vi "Toggle.vi"(1 "Input":bool, 2 "Case":enum16{"Only Press", "Toggle"}(ring)) -> (0 "Output":bool)   [LabVIEW 2014]
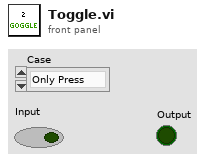
[diagram p1: front panel]
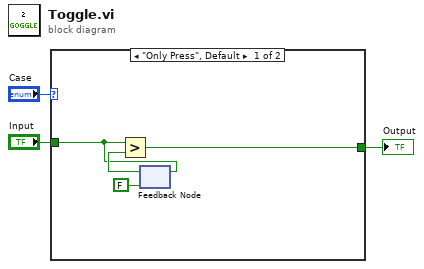
[diagram p0: block diagram]
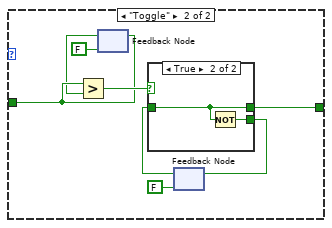
[diagram p2: hidden frame]
diagram:
  n1 = case shown="\"Only Press\", Default" "Case" {
    tunnel: "Input" -> [w5 w12]
    tunnel: [w4 w8] -> w1
    frame "Only Press", Default {
      n2 = feedback #1(FALSE ("A")) -> (w6:bool)
      n3 = Greater?(x=w5, y=w6) -> (0:w4:bool)
      n4 = feedback-in #1(w5) -> ()
    }
    frame "Toggle" {
      n5 = feedback #2(FALSE ("Input")) -> (w11:bool)
      n6 = Greater?(x=w12, y=w11) -> (0:w13:bool)
      n7 = feedback-in #2(w12) -> ()
      n8 = feedback #3(FALSE ("A")) -> (w15:bool)
      n9 = case shown="True" w13 {
        tunnel: w15 -> [w16 w17]
        tunnel: [w16 w18] -> w9
        tunnel: [w16 w17] -> w8
        frame False {
        }
        frame True {
          n10 = Not(x=w17) -> (.not. x?=w18:bool)
        }
      }
      n11 = feedback-in #3(w9) -> ()
    }
  }
  "Output" <- w1
